vi "Filter Wheel Messenger.vi"(0 "FW Notifier":string, 2 "Actions":T1, 11 "Set Position":u8) -> (15 "Current Position":u8)   [LabVIEW 2016]
uses:
  Thorlabs/FW102C/FW102C Type Defs/FW102C Actions.ctl
  FW Type Defs/FW Notifier Type.ctl
panel:
  in  "Exit While Busy?":bool
  out "FW Notifier (Dup)":string
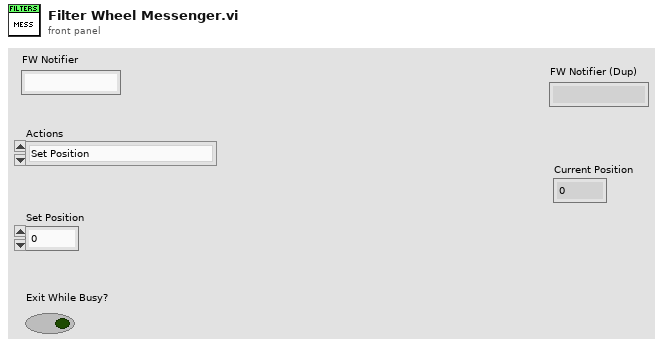
[diagram p1: front panel]
types:
  T1 = typedef "FW102C Actions.ctl" = enum16{"Set Position", "Get Position", "Set Speed", "Quit"}
  T2 = typedef "FW Notifier Type.ctl" = cluster{"Actions":T1, "Set Position":u8, "Actual Position":u8, "Speed":dbl, "Received":bool}
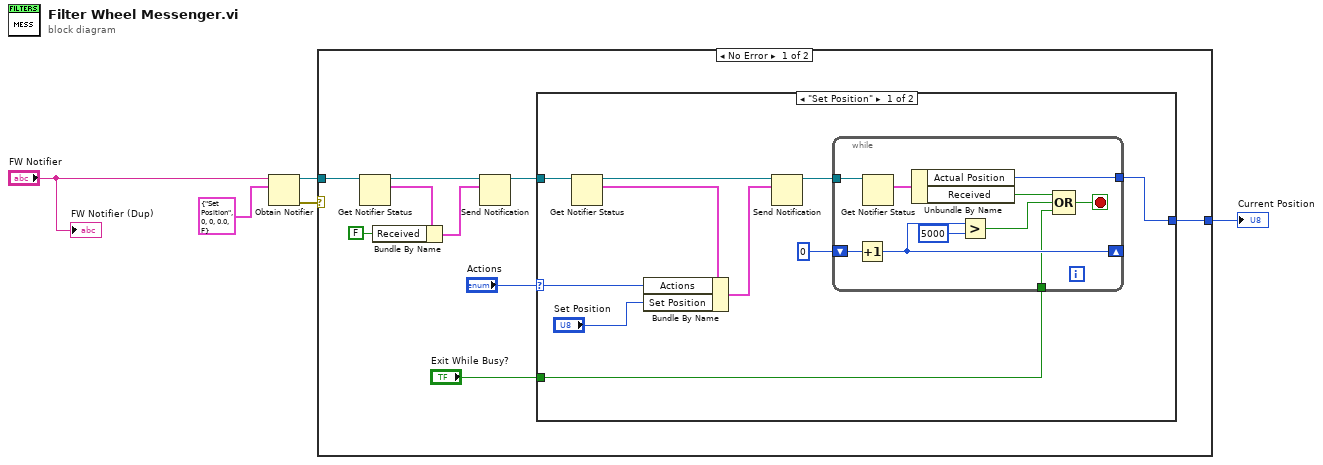
[diagram p0: block diagram]
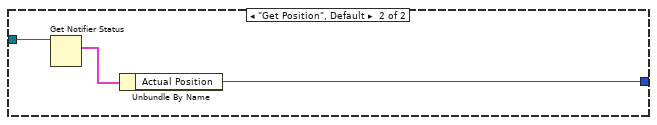
[diagram p2: hidden frame]
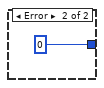
[diagram p3: hidden frame]
diagram:
  n1 = Obtain Notifier(name (unnamed)="FW Notifier", notification data type=T2 {"Actions"=enum."Set Position", "Set Position"=0, "Actual Position"=0, "Speed"=0.0, "Received"=FALSE} ("FW102C Note Type")) -> (notifier out=w2:refnum<notifier>, error out=w3:errorcluster)  [unwired: 2 in, 1 out]
  n2 = case shown="No Error" w3 {
    tunnel: w2 -> [w11 _]
    tunnel: [w6 u8 0 ("Actual Position")] -> w1
    frame No Error {
      n3 = Get Notifier Status(notifier=w11) -> (notifier out=w12:refnum<notifier>, current notification=w9:T2)  [unwired: 1 in, 3 out]
      n4 = Bundle By Name(cluster=w9, "Received"=FALSE) -> (w7:T2)
      n5 = Send Notification(notification=w7, notifier=w12) -> (notifier out=w10:refnum<notifier>)  [unwired: 1 in, 1 out]
      n6 = case shown="\"Set Position\"" "Actions" {
        selector: "Actions" -> [w21 _]
        tunnel: w10 -> [w24 w37]
        tunnel: [w15 w35] -> w6
        tunnel: "Exit While Busy?" -> [w16 _]
        frame "Set Position" {
          n7 = Get Notifier Status(notifier=w24) -> (notifier out=w23:refnum<notifier>, current notification=w22:T2)  [unwired: 1 in, 3 out]
          n8 = Bundle By Name(cluster=w22, "Actions"=w21, "Set Position"="Set Position") -> (w19:T2)
          n9 = Send Notification(notification=w19, notifier=w23) -> (notifier out=w18:refnum<notifier>)  [unwired: 1 in, 1 out]
          n10 = while {
            tunnel: w18 -> [w34]
            shift-right: [w29] -> _
            shift-left: u16 0 -> [w30]
            tunnel: [w26] -> w15
            tunnel: w16 -> [w25]
            stop <- w31 stop-if-true
            n11 = Increment(x=w30) -> (x+1=w29:u16)
            n12 = Get Notifier Status(notifier=w34) -> (current notification=w33:T2)  [unwired: 1 in, 4 out]
            n13 = Unbundle By Name(w33) -> ("Actual Position"=w26:u8, "Received"=w32:bool)
            n14 = Greater?(x=w29, y=u16 5000) -> (0:w27:bool)
            n15 = Compound Arithmetic op=OR(w32, w27, w25) -> (w31:bool)
          }
        }
        frame "Get Position", Default {
          n16 = Get Notifier Status(notifier=w37) -> (current notification=w36:T2)  [unwired: 1 in, 4 out]
          n17 = Unbundle By Name(w36) -> ("Actual Position"=w35:u8)
        }
      }
    }
    frame Error {
    }
  }
  "Current Position" <- w1
  "FW Notifier (Dup)" <- "FW Notifier"
